vi "Data.Result Attribute Look Up Result Code.vi"(4 "Limits":variant, 6 "error in":errorcluster, 7 "Attribute":T1 {"Status" items=["LOG", "PASS", "FAIL", "ERROR"]}) -> (2 "Attribute Out":T1 {"Status" items=["LOG", "PASS", "FAIL", "ERROR"]})   [LabVIEW 2024, in "EQMF.lvlib" / "Data.lvlib"]
uses:
  Data.lvlib
  TypeDefs/Data.Result Attribute.ctl
  TypeDefs/Data.Result Item Status.ctl
  TypeDefs/Data.Result Limit Definition.ctl
  TypeDefs/Data.Result Numeric Limit Type.ctl
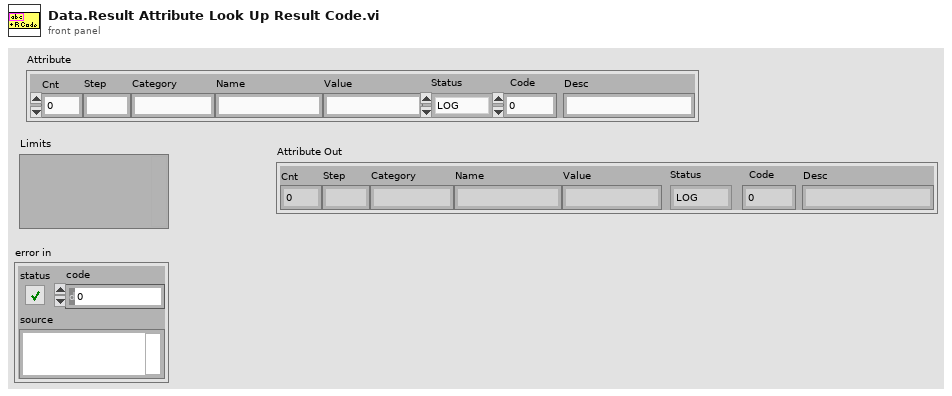
[diagram p1: front panel]
types:
  T1 = typedef "EQMF.lvlib/Data.lvlib/Data.Result Attribute.ctl" = cluster{"Cnt":i32, "Step":string, "Category":string, "Name":string, "Value":string, "Status":T2, "Code":i32, "Desc":string}
  T2 = typedef "EQMF.lvlib/Data.lvlib/Data.Result Item Status.ctl" = i32
  T3 = typedef "EQMF.lvlib/Data.lvlib/Data.Result Limit Definition.ctl" = cluster{"Name":string, "LimType":T4, "LL":dbl, "UL":dbl, "Units":string, "FailCode":i32, "FailDesc":string}
  T4 = typedef "EQMF.lvlib/Data.lvlib/Data.Result Numeric Limit Type.ctl" = enum16{"None", "EQ", "NE", "GT", "LT", "GE", "LE", "GTLT", "GELE", "GELT", "GTLE", "LTGT", "LEGE", "LEGT", "LTGE"}
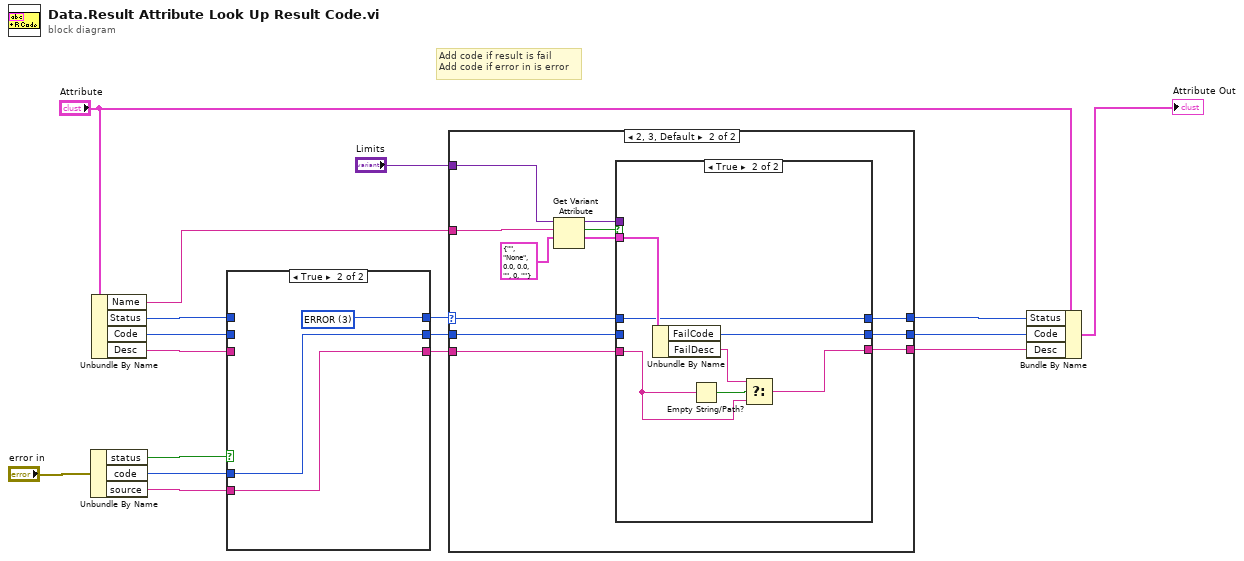
[diagram p0: block diagram]
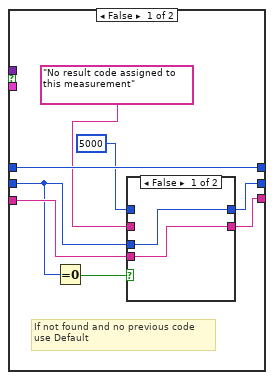
[diagram p3: hidden frame]
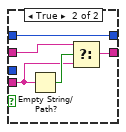
[diagram p4: hidden frame]
diagram:
  # "Add code if result is fail\nAdd code if error in is error"
  n1 = Unbundle By Name("error in") -> ("status"=w14:bool, "code"=w12:i32, "source"=w11:string)
  n2 = Unbundle By Name("Attribute") -> ("Name"=w6:string, "Status"=w13:T2, "Code"=w3:i32, "Desc"=w2:string)
  n3 = case shown="True" w14 {
    tunnel: [w20 w21] -> w1
    tunnel: w13 -> [w20 _]
    tunnel: w12 -> [_ w23]
    tunnel: [w19 w23] -> w9
    tunnel: w11 -> [_ w22]
    tunnel: [w18 w22] -> w8
    tunnel: w3 -> [w19 _]
    tunnel: w2 -> [w18 _]
    frame False {
    }
    frame True {
      w21 = T2 3 items=["LOG", "PASS", "FAIL", "ERROR"] ("Status")
    }
  }
  n4 = case shown="2, 3, Default" w1 {
    selector: w1 -> [w26 w31]
    tunnel: [w26 w30] -> w10
    tunnel: w9 -> [w25 w29]
    tunnel: w8 -> [w24 w28]
    tunnel: [w25 w34] -> w7
    tunnel: w6 -> [_ w35]
    tunnel: [w24 w33] -> w5
    tunnel: "Limits" -> [_ w32]
    frame 0, 1 {
      # "Log or PASS\nNo fail code"
    }
    frame 2, 3, Default {
      n5 = Get Variant Attribute(Variant=w32, name=w35, default value (empty Variant)=T3 {"Name"="", "LimType"=enum."None", "LL"=0.0, "UL"=0.0, "Units"="", "FailCode"=0, "FailDesc"=""} ("KATE_Lib.lvlib:Data.lvlib:Data.Result Limit Definition")) -> (duplicate Variant=w37:variant, found=w38:bool, value=w36:T3)  [unwired: 1 in, 1 out]
      n6 = case shown="True" w38 {
        tunnel: w37 -> [_ _]
        tunnel: w36 -> [_ w59]
        tunnel: [w42 w60] -> w34
        tunnel: [w41 w54] -> w33
        tunnel: w31 -> [w46 w58]
        tunnel: [w46 w58] -> w30
        tunnel: w29 -> [w43 _]
        tunnel: w28 -> [w44 w55]
        frame False {
          # "If not found and no previous code\nuse Default"
          n7 = Equal To 0?(x=w43) -> (x = 0?=w45:bool)
          n8 = case shown="False" w45 {
            tunnel: w44 -> [w47 w49]
            tunnel: w43 -> [w48 _]
            tunnel: 5000 ("Code") -> [_ w53]
            tunnel: "No result code assigned to this measurement" ("Desc") -> [_ w51]
            tunnel: [w48 w53] -> w42
            tunnel: [w47 w50] -> w41
            frame False {
            }
            frame True {
              n9 = Empty String/Path?(string/path=w49) -> (empty?=w52:bool)
              n10 = Select(t=w51, s=w52, f=w49) -> (s? t:f=w50:string)
            }
          }
        }
        frame True {
          n11 = Unbundle By Name(w59) -> ("FailCode"=w60:i32, "FailDesc"=w56:string)
          n12 = Empty String/Path?(string/path=w55) -> (empty?=w57:bool)
          n13 = Select(t=w56, s=w57, f=w55) -> (s? t:f=w54:string)
        }
      }
    }
  }
  n14 = Bundle By Name(cluster="Attribute", "Status"=w10, "Code"=w7, "Desc"=w5) -> (→"Attribute Out":T1)
